vi "Vision Research Phantom Series PhFile PhGetSaveCinePath.vi"(1 "CH in":u64=1, 5 "Error In (no error)":errorcluster) -> (15 "CH out":u64=1, 17 "Success":bool, 19 "Error Out":errorcluster)   [LabVIEW 2013, in "VRI.lvlib"]
doc: "PhFile.dll\n\nPhGetSaveCinePath\nBOOL PhGetSaveCinePath(CINEHANDLE CH);\n\nParameters Description\nCH (in, out) Handle of the cine to be saved.\nReturn TRUE - The operation has succeeded. The user ended the\n dialog with OK.\n FALSE - The operation has been canceled. The user\n ended the dialog with CANCEL.\nComments Allows the user to select a folder where the result(s) of\n converting one or multiple source files will be stored."
uses:
  VRI.lvlib
  Phantom DLLs/PhFile.dll
panel:
  # "For instructions on the use of this VI, press Ctrl+H to display the help window and move the mouse over the icon, controls, and indicators"
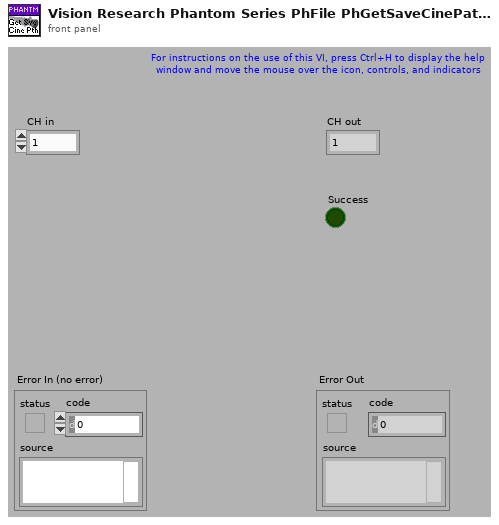
[diagram p1: front panel]
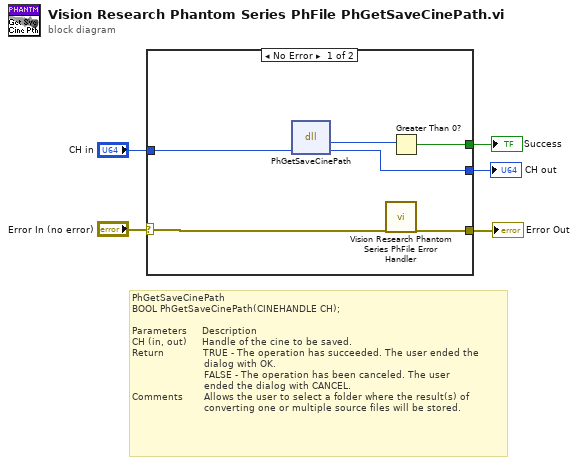
[diagram p0: block diagram]
diagram:
  # "PhGetSaveCinePath\nBOOL PhGetSaveCinePath(CINEHANDLE CH);\n\nParameters     Description\nCH (in, out)     Handle of the cine to be saved.\nReturn             TRUE - The operation has succeeded. The user ended the\n                        dialog with OK.\n                        FALSE - The operation has been canceled. The user\n                        ended the dialog with CANCEL.\nComments       Allows the user to select a folder where the result(s) of\n                        converting one or multiple source files will be stored."
  n1 = case shown="No Error" "Error In (no error)" {
    selector: "Error In (no error)" -> [w11 w13]
    tunnel: [w10 w13] -> w4
    tunnel: "CH in" -> [w9 w12]
    tunnel: [w8 w12] -> w2
    tunnel: [w7 _] -> w1
    frame No Error {
      n2 = dll-call lib="C:/Projects/SDK/32-bit/Vision Research Phantom Series Labview Driver/Phantom DLLs/PhFile.dll" fn="PhGetSaveCinePath"("CH"=w9) -> ("return type"=w6:i32, "CH"=w8:u64)  [unwired: 3 in, 2 out]
      n3 = call "Vision Research Phantom Series PhFile Error Handler.vi"("Error In (no error)"=w11) -> ("Error Out"=w10:errorcluster)  [unwired: 1 in, 17 out]
      n4 = Greater Than 0?(x=w6) -> (x > 0?=w7:bool)
    }
    frame Error {
    }
  }
  "Error Out" <- w4
  "CH out" <- w2
  "Success" <- w1
